vi "initvar.vi"   [LabVIEW 2015]
uses:
  G_ALL.vi
  G_SEN.vi
  G_LCM.vi
types:
  T1 = cluster{"hash":i64, "sys time":i64, "time":dbl, "x":dbl, "y":dbl, "h":dbl, "numSV":i32, "postype":i32, "lag":i32, "hordev":dbl, "lat":dbl, "lon":dbl, "hgt":dbl, "map_idx":i32}
  T2 = cluster{"C_Wheel base":dbl, "ratio_steer":dbl, "Overall width":dbl, "af":dbl, "turn radius":dbl, "eval":dbl, "ap":dbl, "an":dbl, "Vmax":dbl, "mu":dbl, "Vlast":dbl}
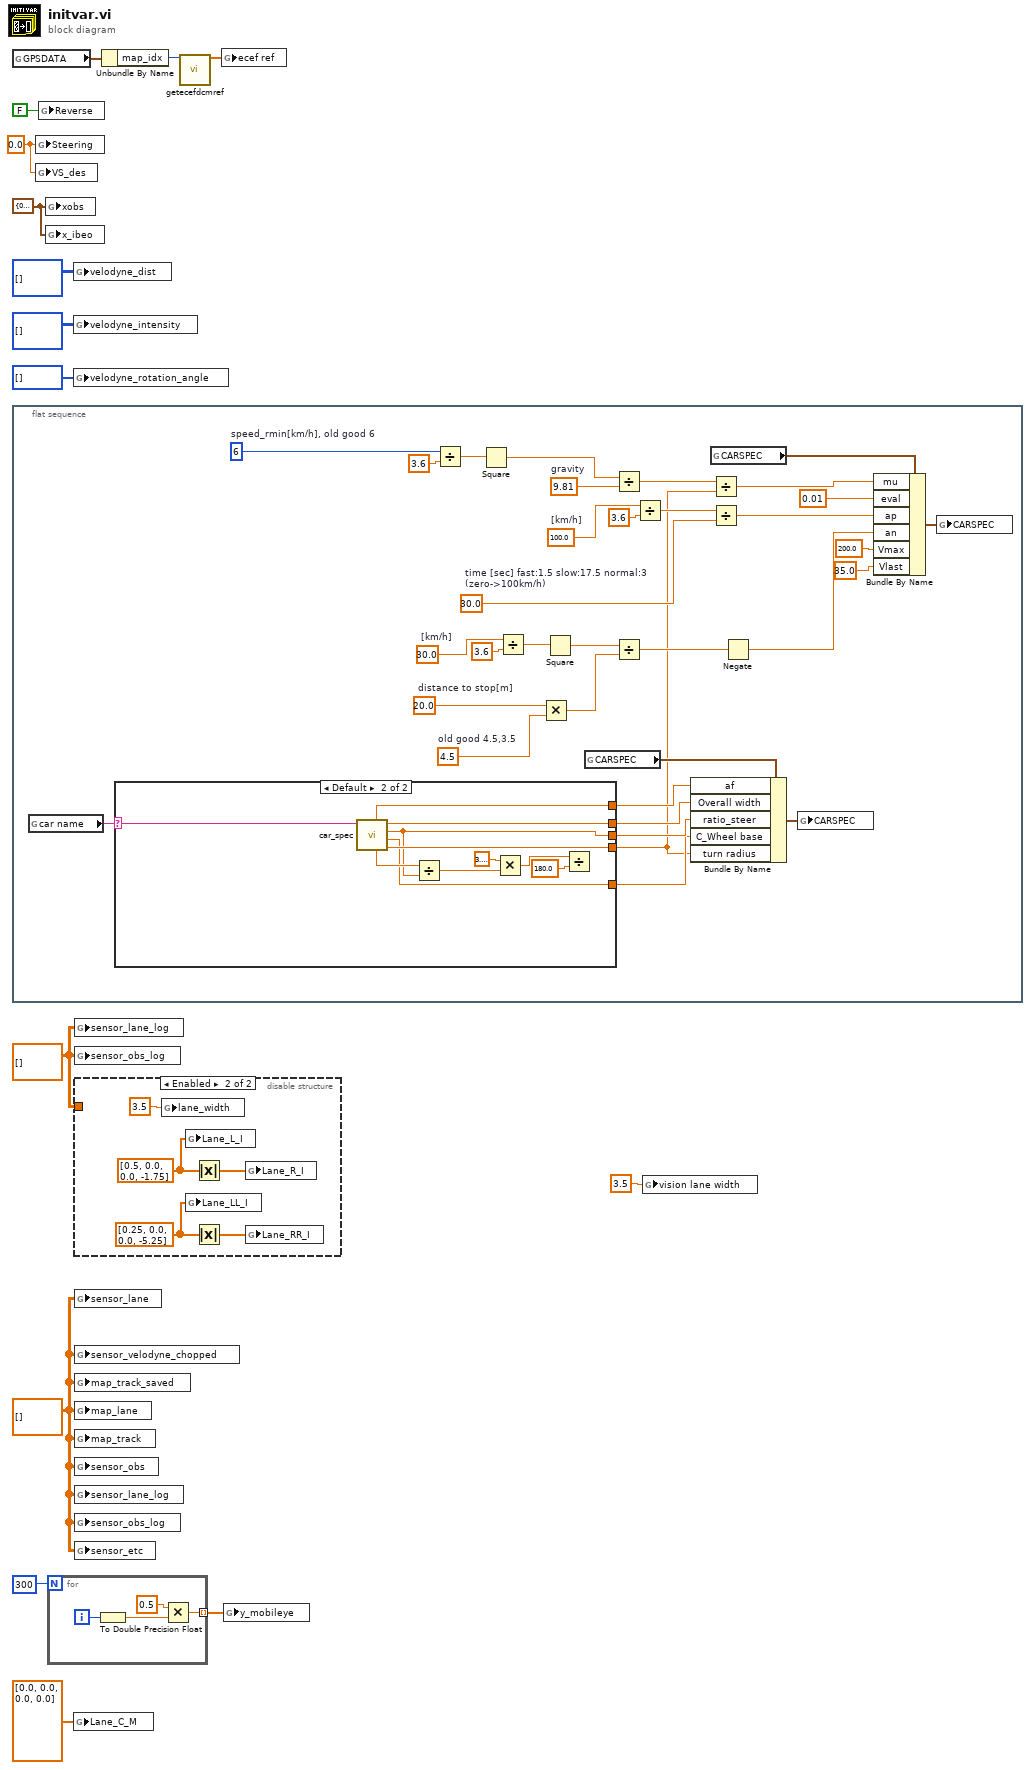
[diagram p0: block diagram]
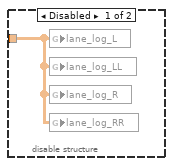
[diagram p2: hidden frame]
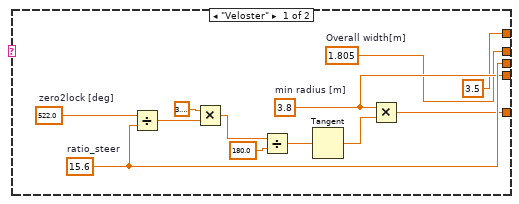
[diagram p3: hidden frame]
diagram:
  w3 = cluster{"idx":i32, "x":dbl, "y":dbl, "h":dbl} {"idx"=0, "x"=0.0, "y"=0.0, "h"=0.0} ("xobs")
  w2 = 0.0
  w6 = dbl[][] [] ("sensor_car")
  w15 = dbl[][] [] ("sensor_obs")
  n1 = global read "G_ALL.vi" "GPSDATA"() -> (w8:T1)
  n2 = flat-sequence {
    frame #0 {
      w33 = 9.81  # gravity
      w37 = 6  # speed_rmin[km/h], old good 6
      w41 = 100.0  # [km/h]
      w38 = 30.0  # time [sec] fast:1.5 slow:17.5 normal:3 (zero->100km/h)
      w45 = 4.5  # old good 4.5,3.5
      w46 = 20.0  # distance to stop[m]
      w48 = 30.0  # [km/h]
      n3 = global read "G_LCM.vi" "car name"() -> (w31:string)
      n4 = case shown="Default" w31 {
        selector: w31 -> [_ w72]
        tunnel: [w56 w65] -> w26
        tunnel: [w53 w71] -> w18
        tunnel: [w52 w64] -> w25
        tunnel: [w51 w63] -> w27
        tunnel: [3.5 ("af") w62] -> w28
        frame "Veloster" {
          w51 = 1.805  # Overall width[m]
          w53 = 3.8  # min radius [m]
          w57 = 522.0  # zero2lock [deg]
          w56 = 15.6  # ratio_steer
          n5 = Divide(x=w57, y=w56) -> (x/y=w61:dbl)
          n6 = Multiply(x=3.141592653589793, y=w61) -> (x*y=w59:dbl)
          n7 = Divide(x=w59, y=180.0) -> (x/y=w55:dbl)
          n8 = Tangent(1:w55) -> (0:w54:dbl)
          n9 = Multiply(x=w53, y=w54) -> (x*y=w52:dbl)
        }
        frame Default {
          n10 = call "car_spec.vi"("Car_name"=w72) -> ("turn radius"=w71:dbl, "wheel base"=w64:dbl, "ratio"=w65:dbl, "overall width"=w63:dbl, "maximum steering angle [deg]"=w66:dbl, "af"=w62:dbl)  [unwired: 5 in]
          n11 = Divide(x=w66, y=w65) -> (x/y=w70:dbl)
          n12 = Multiply(x=3.141592653589793, y=w70) -> (x*y=w68:dbl)
          n13 = Divide(x=w68, y=180.0) -> ()  [unwired: 1 out]
        }
      }
      n14 = Divide(x=w37, y=3.6) -> (x/y=w35:dbl)
      n15 = Square(x=w35) -> (x^2=w34:dbl)
      n16 = Divide(x=w48, y=3.6) -> (x/y=w47:dbl)
      n17 = Multiply(x=w46, y=w45) -> (x*y=w44:dbl)
      n18 = Square(x=w47) -> (x^2=w43:dbl)
      n19 = global read "G_ALL.vi" "CARSPEC"() -> (w30:T2)
      n20 = Divide(x=w34, y=w33) -> (x/y=w32:dbl)
      n21 = Divide(x=w43, y=w44) -> (x/y=w42:dbl)
      n22 = Divide(x=w41, y=3.6) -> (x/y=w39:dbl)
      n23 = Bundle By Name(cluster=w30, "af"=w28, "Overall width"=w27, "ratio_steer"=w26, "C_Wheel base"=w25, "turn radius"=w18) -> (w29:T2)
      n24 = global read "G_ALL.vi" "CARSPEC"() -> (w24:T2)
      n25 = Divide(x=w32, y=w18) -> (x/y=w17:dbl)
      n26 = Divide(x=w39, y=w38) -> (x/y=w20:dbl)
      n27 = Negate(x=w42) -> (-x=w21:dbl)
      n28 = global write "G_ALL.vi" "CARSPEC"(w29) -> ()
      n29 = Bundle By Name(cluster=w24, "mu"=w17, "eval"=0.01, "ap"=w20, "an"=w21, "Vmax"=200.0, "Vlast"=35.0) -> (w23:T2)
      n30 = global write "G_ALL.vi" "CARSPEC"(w23) -> ()
    }
  }
  n31 = global write "G_ALL.vi" "Steering"(w2) -> ()
  n32 = global write "G_ALL.vi" "VS_des"(w2) -> ()
  n33 = global write "G_ALL.vi" "Reverse"(FALSE ("Reverse")) -> ()
  n34 = global write "G_ALL.vi" "xobs"(w3) -> ()
  n35 = global write "G_ALL.vi" "x_ibeo"(w3) -> ()
  n36 = for {
    N: 300 -> [_]
    tunnel: [w73] -> w10 mode=indexing
    i -> [w76]
    n37 = To Double Precision Float(number=w76) -> (double precision float=w75:dbl)
    n38 = Multiply(x=0.5, y=w75) -> (x*y=w73:dbl)
  }
  n39 = global write "G_SEN.vi" "velodyne_dist"(u16[][] [] ("velodyne_dist")) -> ()
  n40 = global write "G_SEN.vi" "velodyne_intensity"(u8[][] [] ("velodyne_intensity")) -> ()
  n41 = global write "G_SEN.vi" "velodyne_rotation_angle"(u16[] [] ("velodyne_rotation_angle")) -> ()
  n42 = global write "G_SEN.vi" "Lane_C_M"(dbl[] [0.0, 0.0, 0.0, 0.0] ("Lane_C_M")) -> ()
  n43 = global write "G_SEN.vi" "sensor_lane_log"(w15) -> ()
  n44 = global write "G_SEN.vi" "sensor_obs_log"(w15) -> ()
  n45 = disable-structure shown="Enabled" {
    disable-tunnel: w15 -> [w77 _]
    frame Disabled {
      n46 = global write "G_SEN.vi" "lane_log_L"(w77) -> ()
      n47 = global write "G_SEN.vi" "lane_log_LL"(w77) -> ()
      n48 = global write "G_SEN.vi" "lane_log_R"(w77) -> ()
      n49 = global write "G_SEN.vi" "lane_log_RR"(w77) -> ()
    }
    frame Enabled {
      w78 = dbl[] [0.25, 0.0, 0.0, -5.25] ("Lane_L_I")
      w81 = dbl[] [0.5, 0.0, 0.0, -1.75] ("Lane_L_I")
      n50 = global write "G_SEN.vi" "lane_width"(3.5 ("lane_width")) -> ()
      n51 = global write "G_SEN.vi" "Lane_L_I"(w81) -> ()
      n52 = global write "G_SEN.vi" "Lane_LL_I"(w78) -> ()
      n53 = Absolute Value(x=w81) -> (abs(x)=w80:dbl[])
      n54 = Absolute Value(x=w78) -> (abs(x)=w79:dbl[])
      n55 = global write "G_SEN.vi" "Lane_R_I"(w80) -> ()
      n56 = global write "G_SEN.vi" "Lane_RR_I"(w79) -> ()
    }
  }
  n57 = global write "G_SEN.vi" "sensor_lane"(w6) -> ()
  n58 = global write "G_SEN.vi" "sensor_velodyne_chopped"(w6) -> ()
  n59 = global write "G_ALL.vi" "map_track_saved"(w6) -> ()
  n60 = global write "G_SEN.vi" "map_lane"(w6) -> ()
  n61 = global write "G_ALL.vi" "map_track"(w6) -> ()
  n62 = global write "G_SEN.vi" "sensor_obs"(w6) -> ()
  n63 = global write "G_SEN.vi" "sensor_lane_log"(w6) -> ()
  n64 = global write "G_SEN.vi" "sensor_obs_log"(w6) -> ()
  n65 = global write "G_SEN.vi" "sensor_etc"(w6) -> ()
  n66 = Unbundle By Name(w8) -> ("map_idx"=w7:i32)
  n67 = call "getecefdcmref.vi"("map name"=w7) -> ("XYZ"=w5:dbl[])  [unwired: 10 in, 4 out]
  n68 = global write "G_ALL.vi" "ecef ref"(w5) -> ()
  n69 = global write "G_SEN.vi" "y_mobileye"(w10) -> ()
  n70 = global write "G_SEN.vi" "vision lane width"(3.5 ("vision lane width")) -> ()
